vi "Eje X_MAINmodificado.vi"() -> ()   [LabVIEW 2016]
doc: "Desarrollo con funcion de DAQ 6008/6009 para mover eje x de GAlvoescanner."
uses:
  Controles/Estados.ctl
  <vilib>/DAQmx/write.llb/DAQmx Write (Analog DBL 1Chan 1Samp).vi
  <vilib>/DAQmx/miscellaneous.llb/DAQmx Fill In Error Info.vi
panel:
  in  "# Ciclos":u16=1 min=1 max=20000 step=1
  out "Volt":dbl caption="Voltaje"
  in  "ms to wait":u32=7 min=7 max=1000 step=1
  out "Error Out":errorcluster
  in  "Go":bool caption="Ir"
  in  "Angle":dbl caption="Ángulo" min=-10.0 max=10.0 step=0.01
  in  "Step_A":dbl=0.01 caption="Paso ángulo" min=0.001 max=10.0 step=0.001
  in  "Stop_A":dbl caption="Ángulo final" min=-5.0 max=5.0 step=0.05
  in  "Start_A":dbl caption="Ángulo inicial" min=-5.0 max=5.0 step=0.05
  in  "Home":bool
  in  "Salir":bool
  in  "Start":bool
  # "Desarrollo: Jhony Turizo\nAbril 2016"
  # "Control GalvoScanner V2.0"
  # "Resolucion teorica\n0.014°"
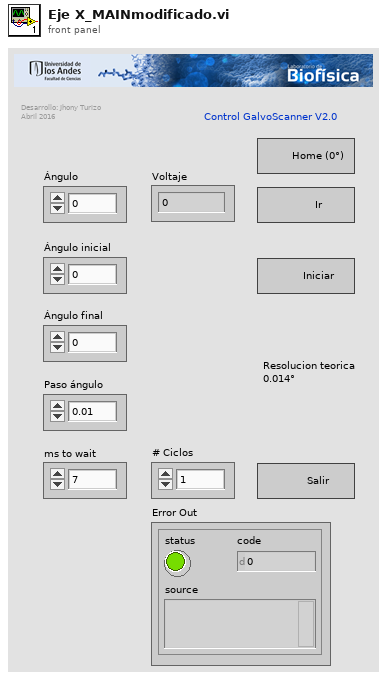
[diagram p1: front panel]
types:
  T1 = typedef "Estados.ctl" = enum16{"Scanning", "Rampa-to+", "Rampa+to-", "Salir"}
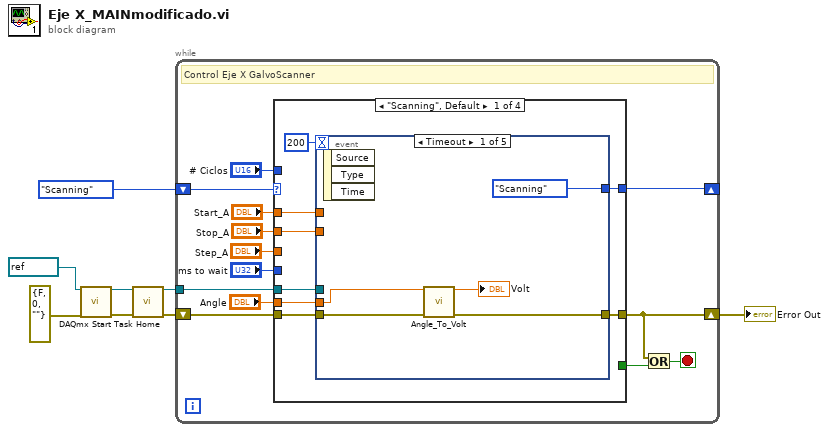
[diagram p0: block diagram]
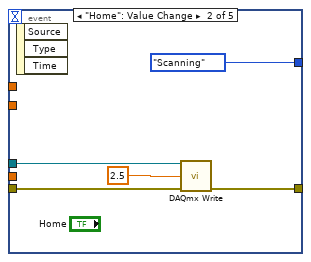
[diagram p2: hidden frame]
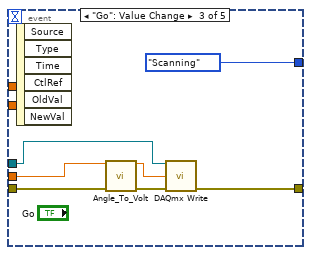
[diagram p3: hidden frame]
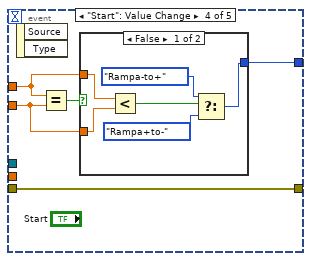
[diagram p4: hidden frame]
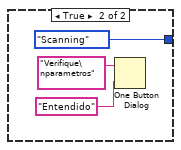
[diagram p5: hidden frame]
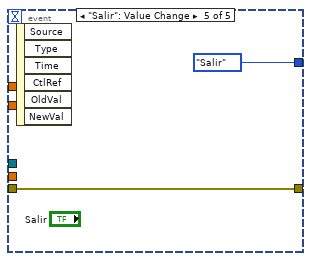
[diagram p6: hidden frame]
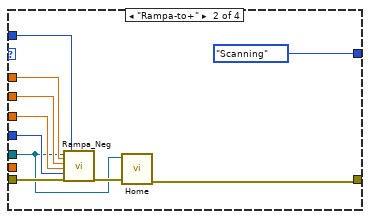
[diagram p7: hidden frame]
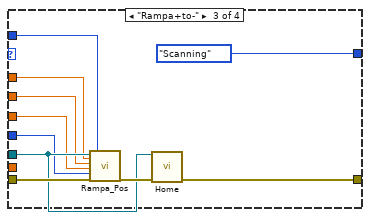
[diagram p8: hidden frame]
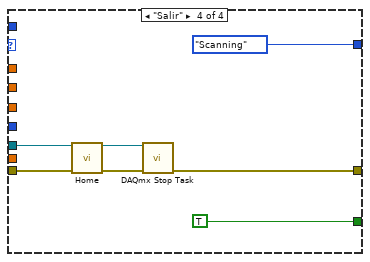
[diagram p9: hidden frame]
diagram:
  n1 = call <vilib>:"DAQmx Start Task.vi"("task/channels in"=refnum<k21> "EjeX", "error in"=errorcluster {"status"=FALSE, "code"=0, "source"=""}) -> ("task out"=w3:refnum<k21>, "error out"=w4:errorcluster)  [unwired: 12 in]
  n2 = call "Home.vi"("Refnum in"=w3, "error in (no error)"=w4) -> ("Refnum out"=w2:refnum<k21>, "error out"=w1:errorcluster)  [unwired: 12 in]
  n3 = while {
    tunnel: w2 -> [w16]
    shift-right: [w15] -> _
    shift-left: Estados."Scanning" -> [w21]
    shift-right: [w18] -> w5
    shift-left: w1 -> [w20]
    stop <- w19 stop-if-true
    # "Control Eje X GalvoScanner"
    n4 = case shown="\"Scanning\", Default" w21 {
      tunnel: w20 -> [w28 w72 w82 w87]
      tunnel: [w26 w64 w79 w83] -> w18
      tunnel: [_ _ _ TRUE] -> w17
      tunnel: w16 -> [w27 w65 w78 w86]
      tunnel: [w25 Estados."Scanning" Estados."Scanning" Estados."Scanning"] -> w15
      tunnel: "Start_A" -> [w24 w70 w77 _]
      tunnel: "Stop_A" -> [w23 w69 w76 _]
      tunnel: "Step_A" -> [_ w68 w75 _]
      tunnel: "ms to wait" -> [_ w67 w74 _]
      tunnel: "Angle" -> [w22 _ _ _]
      tunnel: "# Ciclos" -> [_ w63 w73 _]
      frame "Scanning", Default {
        n5 = event shown="[0] Timeout" {
          selector: _ -> [_ _ _ _ _]
          dyn-events: _ -> [_ _ _ _ _]
          timeout: 200 -> [_ _ _ _ _]
          tunnel: w28 -> [w33 w39 w44 w50 w62]
          tunnel: w27 -> [_ w38 w43 _ _]
          tunnel: [w32 w37 w46 w50 w62] -> w26
          tunnel: [Estados."Scanning" Estados."Scanning" Estados."Scanning" w47 Estados."Salir"] -> w25
          tunnel: w24 -> [_ _ _ w49 _]
          tunnel: w23 -> [_ _ _ w48 _]
          tunnel: w22 -> [w30 _ w40 _ _]
          event Timeout {
            n6 = event-data() -> ()  [unwired: 1 in, 3 out]
            n7 = call "Angle_To_Volt.vi"("Angulo IN"=w30, "Error In"=w33) -> ("Voltaje OUT"=→"Volt":dbl, "Error Out"=w32:errorcluster)  [unwired: 12 in]
          }
          event "Home": Value Change {
            n8 = event-data() -> ()  [unwired: 1 in, 3 out]
            n9 = call-poly <vilib>:"DAQmx Write.vi"("task/channels in"=w38, "data"=2.5, "error in"=w39) -> ("error out"=w37:errorcluster)  [unwired: 10 in, 2 out]
          }
          event "Go": Value Change {
            n10 = event-data() -> ()  [unwired: 1 in, 6 out]
            n11 = call "Angle_To_Volt.vi"("Angulo IN"=w40, "Error In"=w44) -> ("Voltaje OUT"=w41:dbl, "Error Out"=w42:errorcluster)  [unwired: 12 in]
            n12 = call-poly <vilib>:"DAQmx Write.vi"("task/channels in"=w43, "data"=w41, "error in"=w42) -> ("error out"=w46:errorcluster)  [unwired: 10 in, 2 out]
          }
          event "Start": Value Change {
            n13 = event-data() -> ()  [unwired: 1 in, 2 out]
            n14 = Equal?(x=w49, y=w48) -> (x = y?=w51:bool)
            n15 = case shown="False" w51 {
              tunnel: w49 -> [w57 _]
              tunnel: w48 -> [w56 _]
              tunnel: [w54 Estados."Scanning"] -> w47
              frame False {
                n16 = Less?(x=w57, y=w56) -> (x < y?=w55:bool)
                n17 = Select(t=Estados."Rampa-to+", s=w55, f=Estados."Rampa+to-") -> (s? t:f=w54:T1)
              }
              frame True {
                n18 = One Button Dialog(message="Verifique\nparametros", button name ("OK")="Entendido") -> ()  [unwired: 1 out]
              }
            }
          }
          event "Salir": Value Change {
            n19 = event-data() -> ()  [unwired: 1 in, 6 out]
          }
        }
      }
      frame "Rampa-to+" {
        n20 = call "Rampa_Neg.vi"("task/channels in"=w65, "Start_A"=w70, "Stop_A"=w69, "Step_A"=w68, "ms to wait"=w67, "Error In"=w72, "# Ciclos"=w63) -> ("Error Out"=w66:errorcluster)  [unwired: 12 in]
        n21 = call "Home.vi"("Refnum in"=w65, "error in (no error)"=w66) -> ("error out"=w64:errorcluster)  [unwired: 12 in, 1 out]
      }
      frame "Rampa+to-" {
        n22 = call "Rampa_Pos.vi"("task/channels in"=w78, "Start_A"=w77, "Stop_A"=w76, "Step_A"=w75, "ms to wait"=w74, "Error In"=w82, "# Ciclos"=w73) -> ("Error Out"=w80:errorcluster)  [unwired: 12 in]
        n23 = call "Home.vi"("Refnum in"=w78, "error in (no error)"=w80) -> ("error out"=w79:errorcluster)  [unwired: 12 in, 1 out]
      }
      frame "Salir" {
        n24 = call "Home.vi"("Refnum in"=w86, "error in (no error)"=w87) -> ("Refnum out"=w84:refnum<k21>, "error out"=w85:errorcluster)  [unwired: 12 in]
        n25 = call <vilib>:"DAQmx Stop Task.vi"("task/channels in"=w84, "error in"=w85) -> ("error out"=w83:errorcluster)  [unwired: 12 in, 1 out]
      }
    }
    n26 = Or(x=w18, y=w17) -> (x .or. y?=w19:bool)
  }
  "Error Out" <- w5
